vi "getAdditionalDataXML.vi"(8 "error in (no error)":errorcluster, 11 "RampEvent in":refnum<class "RampEvent.lvclass">) -> (0 "error out":errorcluster, 2 "additionalDataXML":refnum<class "xmlNode.lvclass">, 3 "RampEvent out":refnum<class "RampEvent.lvclass">)   [LabVIEW 2009, in "Tools.lvlib" / "Scripting.lvlib" / "RampEvent.lvclass"]
uses:
  RampEvent.lvclass
  xmlNode/xmlNode.lvclass
  RampEvent.lvclass/RampEvent.ctl
  ScriptEvent.lvclass
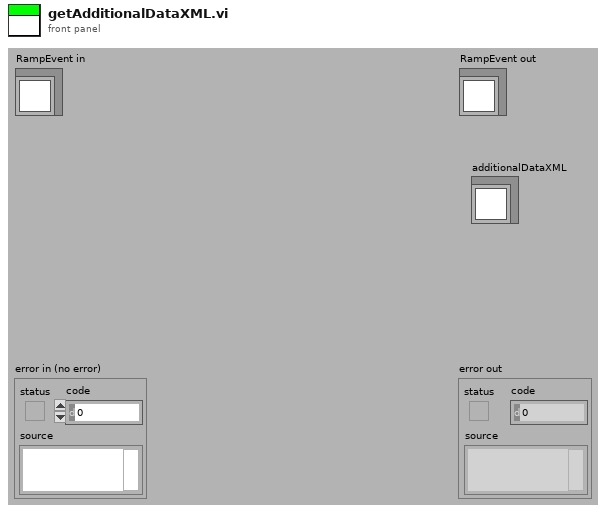
[diagram p1: front panel]
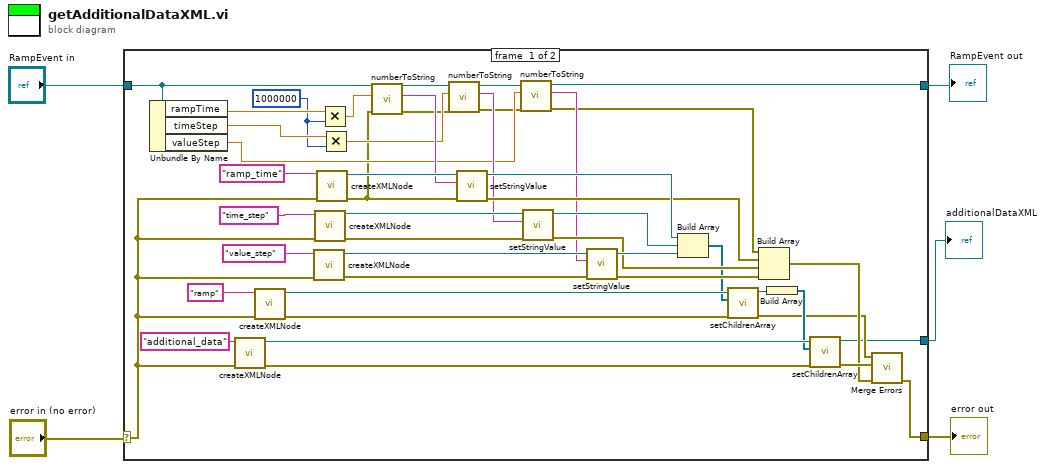
[diagram p0: block diagram]
diagram:
  n1 = case shown="No Error" "error in (no error)" {
    selector: "error in (no error)" -> [w47 w52]
    tunnel: "RampEvent in" -> [w19 w53]
    tunnel: [w12 w53] -> w3
    tunnel: [w23 w52] -> w2
    tunnel: [w22 _] -> w1
    frame #0 {
      w44 = 1000000
      n2 = Unbundle By Name(w19) -> ("rampTime"=w46:dbl, "timeStep"=w45:dbl, "valueStep"=w10:dbl)
      n3 = call "createXMLNode.vi"("error in (no error)"=w47, "name"="additional_data") -> ("error out"=w20:errorcluster, "xmlNode out"=w29:refnum<class "xmlNode.lvclass">)  [unwired: 8 in]
      n4 = call "createXMLNode.vi"("error in (no error)"=w47, "name"="ramp") -> ("error out"=w30:errorcluster, "xmlNode out"=w32:refnum<class "xmlNode.lvclass">)  [unwired: 8 in]
      n5 = call "createXMLNode.vi"("error in (no error)"=w47, "name"="value_step") -> ("error out"=w39:errorcluster, "xmlNode out"=w40:refnum<class "xmlNode.lvclass">)  [unwired: 8 in]
      n6 = call "createXMLNode.vi"("error in (no error)"=w47, "name"="time_step") -> ("error out"=w41:errorcluster, "xmlNode out"=w42:refnum<class "xmlNode.lvclass">)  [unwired: 8 in]
      n7 = call "createXMLNode.vi"("error in (no error)"=w47, "name"="ramp_time") -> ("error out"=w6:errorcluster, "xmlNode out"=w43:refnum<class "xmlNode.lvclass">)  [unwired: 8 in]
      n8 = Multiply(x=w46, y=w44) -> (x*y=w18:dbl)
      n9 = Multiply(x=w45, y=w44) -> (x*y=w15:dbl)
      n10 = call "numberToString.vi"("error in (no error)"=w6, "Numeric"=w18, "ScriptEvent in"=w19) -> ("error out"=w9:errorcluster, "String"=w17:string, "ScriptEvent out"=w16:refnum<class "RampEvent.lvclass">)  [unwired: 6 in]
      n11 = call "numberToString.vi"("error in (no error)"=w9, "Numeric"=w15, "ScriptEvent in"=w16) -> ("error out"=w8:errorcluster, "String"=w14:string, "ScriptEvent out"=w13:refnum<class "RampEvent.lvclass">)  [unwired: 6 in]
      n12 = call-dynamic "setStringValue.vi"("error in (no error)"=w6, "stringValue"=w17, "xmlNode.lvclass in"=w43) -> ("error out"=w35:errorcluster, "xmlNode.lvclass out"=w38:refnum<class "xmlNode.lvclass">)  [unwired: 7 in]
      n13 = call "numberToString.vi"("error in (no error)"=w8, "Numeric"=w10, "ScriptEvent in"=w13) -> ("error out"=w7:errorcluster, "String"=w11:string, "ScriptEvent out"=w12:refnum<class "RampEvent.lvclass">)  [unwired: 6 in]
      n14 = call-dynamic "setStringValue.vi"("error in (no error)"=w41, "stringValue"=w14, "xmlNode.lvclass in"=w42) -> ("error out"=w34:errorcluster, "xmlNode.lvclass out"=w37:refnum<class "xmlNode.lvclass">)  [unwired: 7 in]
      n15 = call-dynamic "setStringValue.vi"("error in (no error)"=w39, "stringValue"=w11, "xmlNode.lvclass in"=w40) -> ("error out"=w33:errorcluster, "xmlNode.lvclass out"=w36:refnum<class "xmlNode.lvclass">)  [unwired: 7 in]
      n16 = Build Array(w38, w37, w36) -> (w31:refnum<class "xmlNode.lvclass">[])
      n17 = call-dynamic "setChildrenArray.vi"("error in (no error)"=w30, "Children"=w31, "xmlNode.lvclass in"=w32) -> ("error out"=w24:errorcluster, "xmlNode.lvclass out"=w28:refnum<class "xmlNode.lvclass">)  [unwired: 7 in]
      n18 = Build Array(w7, w35, w34, w33) -> (w25:errorcluster[])
      n19 = Build Array(w28) -> (w27:refnum<class "xmlNode.lvclass">[])
      n20 = call-dynamic "setChildrenArray.vi"("error in (no error)"=w20, "Children"=w27, "xmlNode.lvclass in"=w29) -> ("error out"=w26:errorcluster, "xmlNode.lvclass out"=w22:refnum<class "xmlNode.lvclass">)  [unwired: 7 in]
      n21 = call <vilib>:"Merge Errors.vi"("error array in"=w25, "error in 2 (no error)"=w26, "error in 1 (no error)"=w24) -> ("error out"=w23:errorcluster)  [unwired: 4 in]
    }
    frame #1 {
    }
  }
  "error out" <- w2
  "RampEvent out" <- w3
  "additionalDataXML" <- w1
